vi "JSON to LVObject - Unknown Type - Returns Error 1373.vi"() -> ()   [LabVIEW 2017, in "JSON Serializable Serializer Tests.lvlib"]
uses:
  JSON Serializable Serializer Tests.lvlib
  JSON Serializable Serializer/JSON Serializable Serializer.lvclass
  Mock JSON Serializable/Mock JSON Serializable.lvclass
  <vilib>/Utility/error.llb/Error Cluster From Error Code.vi
  <vilib>/addons/_JKI Toolkits/Caraya/classes/Assert/Assert Equal Value_Variant.vi
  <vilib>/ErrorRing/Error Ring.xnode
  <vilib>/addons/_JKI Toolkits/Caraya/classes/Test/Test.lvclass
  <vilib>/addons/_JKI Toolkits/Caraya/classes/Assert/Assert.lvclass
panel:
  out "error out":errorcluster
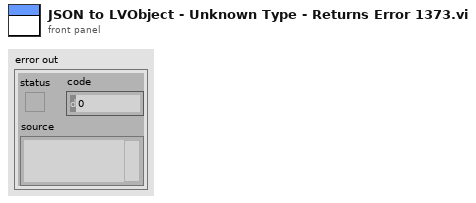
[diagram p1: front panel]
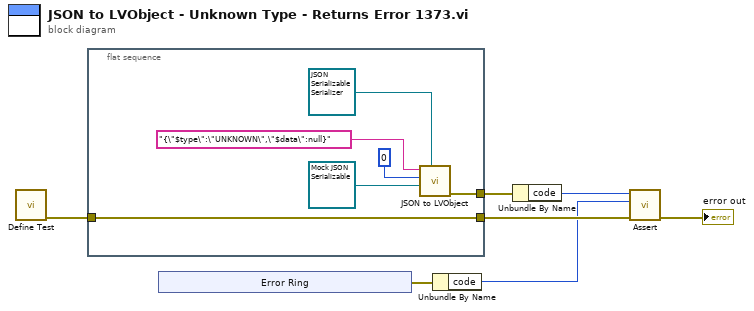
[diagram p0: block diagram]
diagram:
  n1 = call <vilib>:"Define Test.vi"() -> ("error out"=w7:errorcluster)  [unwired: 11 in]
  n2 = flat-sequence {
    tunnel: w7 -> [w8]
    tunnel: [w9] -> w5
    tunnel: [w8] -> w4
    frame #0 {
      n3 = call-dynamic "JSON to LVObject.vi"("JSON Serializer in"=refnum<class "JSON Serializable Serializer.lvclass"> refnum ("JSON Serializer.lvclass"), "Object Type"=refnum<class "Mock JSON Serializable.lvclass"> refnum ("Type"), "Offset"=0, "JSON"="{\"$type\":\"UNKNOWN\",\"$data\":null}") -> ("error out"=w9:errorcluster)  [unwired: 6 in, 1 out]
    }
  }
  n4 = xnode "Error Ring"() -> ("error out"=w3:errorcluster)
  n5 = Unbundle By Name(w3) -> ("code"=w1:i32)
  n6 = Unbundle By Name(w5) -> ("code"=w2:i32)
  n7 = call-poly <vilib>:"Assert.vi"("error in (no error)"=w4, "Y"=w1, "X"=w2) -> ("error out"=→"error out":errorcluster)  [unwired: 8 in]
